vi "Write Data.vi"(6 "Unit ID":u8, 7 "Write Mask":bool[](array[boolean]), 8 "error in (no error)":errorcluster, 9 "Values":dbl[](array[numeric]), 10 "output data access":T1={"Modbus Type"=enum."Input Register", "start"=0, "length"=0, "Channel Data"=[]}, 11 "Modbus Master in":refnum<class "Modbus Master.lvclass">) -> (0 "error out":errorcluster)   [LabVIEW 2020, in "Modbus Master Engine.lvlib"]
uses:
  Modbus Master Engine.lvlib
  Modbus API.lvlibp/API/Master/Modbus Master.lvclass
  C:/Git/Modbus-Custom-Device-v2/Source/Engine/Modbus API.lvlibp/API/Modbus API.lvclass
  Bulk Data Access.ctl
  System Explorer/SubVIs/Modbus Type.ctl
  Shared/Controls/Data Model/Channel.ctl
  <vilib>/NI VeriStand/Custom Device API/Custom Device Channel Type.ctl
  Shared/Controls/Data Model/Mapping.ctl
  Shared/Controls/Data Model/DataType.ctl
  <vilib>/NI VeriStand/Custom Device API/Custom Device Item Ref.ctl
  Shared/Modbus Master Shared.lvlib
  <vilib>/NI VeriStand/Custom Device API/Custom Device API.lvlib
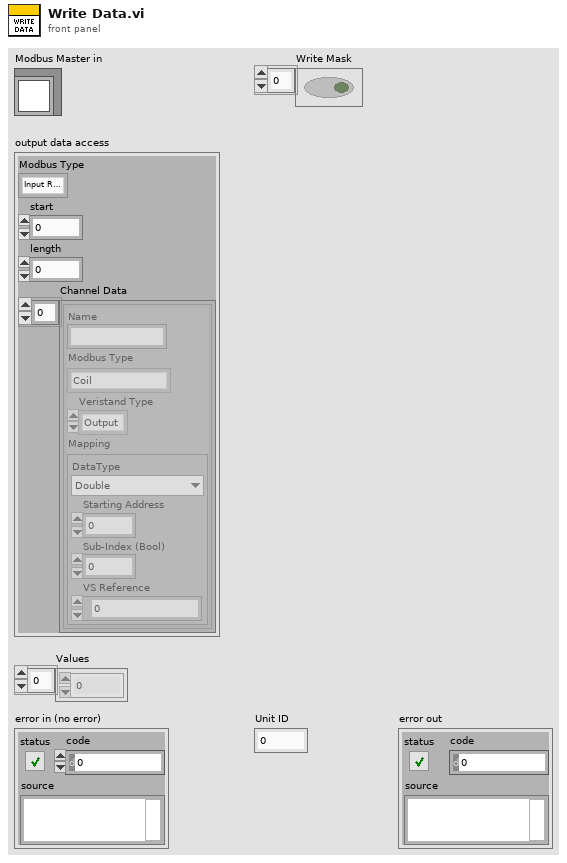
[diagram p1: front panel]
types:
  T1 = typedef "Modbus Master Shared.lvlib/Bulk Data Access.ctl" = cluster{"Modbus Type":T2, "start":u16, "length":u16, "Channel Data":T3[]}
  T2 = typedef "Modbus Master Shared.lvlib/Modbus Type.ctl" = enum16{"Coil", "Discrete Input", "Holding Register", "Input Register"}
  T3 = typedef "Modbus Master Shared.lvlib/Channel.ctl" = cluster{"Name":string, "Modbus Type":T2, "Veristand Type":T4, "Mapping":T5}
  T4 = typedef "Custom Device API.lvlib/Custom Device Channel Type.ctl" = enum16{"Input", "Output"}
  T5 = typedef "Modbus Master Shared.lvlib/Mapping.ctl" = cluster{"DataType":T6, "Starting Address":u16, "Sub-Index (Bool)":u16, "VS Reference":T7}
  T6 = typedef "Modbus Master Shared.lvlib/DataType.ctl" = enum16{"Double", "Single", "I64", "I32", "I16", "I8", "U64", "U32", "U16", "U8", "Boolean"}
  T7 = typedef "Custom Device API.lvlib/Custom Device Item Ref.ctl" = u64
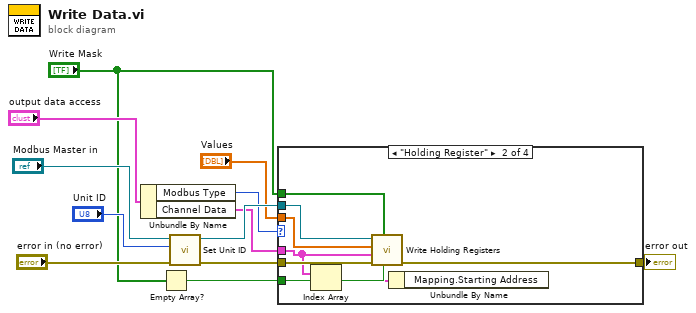
[diagram p0: block diagram]
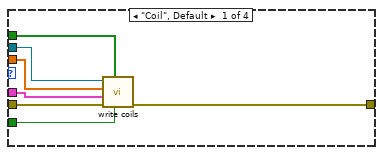
[diagram p2: hidden frame]
diagram:
  n1 = Unbundle By Name("output data access") -> ("Modbus Type"=w4:T2, "Channel Data"=w3:T3[])
  n2 = Empty Array?(array="Write Mask") -> (empty?=w1:bool)
  n3 = call "Set Unit ID.vi"("error in"="error in (no error)", "unit ID"="Unit ID", "Modbus master in"="Modbus Master in") -> ("error out"=w12:errorcluster, "Modbus master out"=w9:refnum<class "Modbus Master.lvclass">)  [unwired: 7 in]
  n4 = case shown="\"Holding Register\"" w4 {
    tunnel: w9 -> [w14 w27 _ _]
    tunnel: [w19 w26 w28 w29] -> w6
    tunnel: w12 -> [w18 w25 w28 w29]
    tunnel: w3 -> [w15 w21 _ _]
    tunnel: "Write Mask" -> [w17 w24 _ _]
    tunnel: "Values" -> [w16 w22 _ _]
    tunnel: w1 -> [w13 w23 _ _]
    frame "Coil", Default {
      n5 = call "write coils.vi"("Ignore Mask?"=w13, "Write Mask"=w17, "error in (no error)"=w18, "Channel Data"=w15, "Values"=w16, "Modbus API.lvlibp:Modbus API"=w14) -> ("error out"=w19:errorcluster)  [unwired: 5 in]
    }
    frame "Holding Register" {
      n6 = Index Array(array=w21) -> (element=w20:T3)  [unwired: 1 in]
      n7 = call "Write Holding Registers.vi"("Ignore Mask?"=w23, "Regs to Write"=w24, "error in (no error)"=w25, "Channel Data"=w21, "Values"=w22, "Modbus API.lvlibp:Modbus API"=w27) -> ("error out"=w26:errorcluster)  [unwired: 5 in]
      n8 = Unbundle By Name(w20) -> ()  [unwired: 1 out]
    }
    frame "Input Register" {
      # "Master can't write\nInput Regs"
    }
    frame "Discrete Input" {
      # "Master can't write\nDiscrete Inputs"
    }
  }
  "error out" <- w6
